vi "DataCNT-Free.vi"(8 "error in (no error)":errorcluster, 11 "DataCNT":T1) -> (0 "error out":errorcluster)   [LabVIEW 2017, in "Data Container.lvlib"]
uses:
  Data Container.lvlib
  TypeDef/Def-DataCNT.ctl
  TypeDef/Def-DataCNT Ico.ctl
  TypeDef/Def-DataCNT DVR.ctl
panel:
  # "Connector Pane"
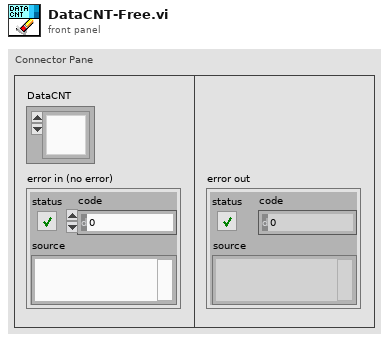
[diagram p1: front panel]
types:
  T1 = typedef "Data Container.lvlib/Def-DataCNT.ctl" = refnum<k1>
  T2 = typedef "Data Container.lvlib/Def-DataCNT DVR.ctl" = refnum<data-value>
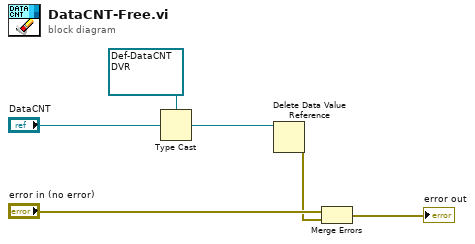
[diagram p0: block diagram]
diagram:
  n1 = Type Cast(type=T2 refnum ("DataCNT Reference"), x="DataCNT") -> (*(type *) &x=w5:T2)
  n2 = Delete Data Value Reference(data value reference=w5) -> (error out=w3:errorcluster)  [unwired: 1 in, 1 out]
  n3 = Merge Errors("error in (no error)", w3) -> (→"error out":errorcluster)
